vi "_Main.vi"   [LabVIEW 2016, in "Controller.lvlib"]
uses:
  Controller.lvlib
  TypeDefs/ENUM_Controller Button List.ctl
  TypeDefs/ENUM_Controller Axis List.ctl
types:
  T1 = typedef "ENUM_Controller Axis List.ctl" = enum16{"Left X", "Left Y", "Left Trigger", "Right Trigger", "Right X", "Right Y"}
  T2 = typedef "ENUM_Controller Button List.ctl" = enum16{"Green A", "Red B", "Blue X", "Yellow Y", "Left Bumper", "Right Bumper", "Back", "Start", "Left Joystick", "Right Joystick"}
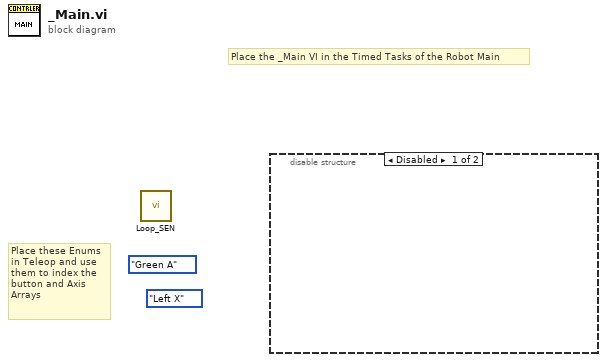
[diagram p0: block diagram]
diagram:
  (unwired) ENUM_Controller_Axis_List."Left X" ("Axes")
  (unwired) ENUM_Controller_Button_List."Green A" ("Buttons")
  # "Place these Enums\nin Teleop and use\nthem to index the \nbutton and Axis\nArrays"
  # "Place the _Main VI in the Timed Tasks of the Robot Main"
  n1 = call "Loop_SEN.vi"() -> ()  [unwired: 12 in]
  n2 = disable-structure shown="Disabled" {
    frame Disabled {
    }
    frame Enabled {
    }
  }
